vi "powermeter-medir.vi"(8 "error in (no error)":errorcluster, 11 "Powermeter":refnum<vi>) -> (0 "error out":errorcluster)   [LabVIEW 2016]
uses:
  controls/powermeter.ctl
  <vilib>/Analysis/NI_AALBase.lvlib
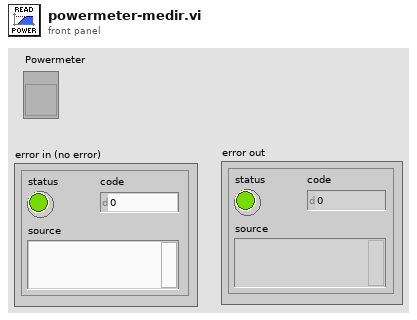
[diagram p1: front panel]
types:
  T1 = typedef "powermeter.ctl" = cluster{"Start":bool, "Serial ":string, "Model":string, "Sensor":string, "Power":dbl, "Density":bool, "Lambda":dbl, "Open":bool, "Save":bool, "reference":refnum<k7>, "hDevice":i32, "Dev. Std.":dbl, "Channel":i16}
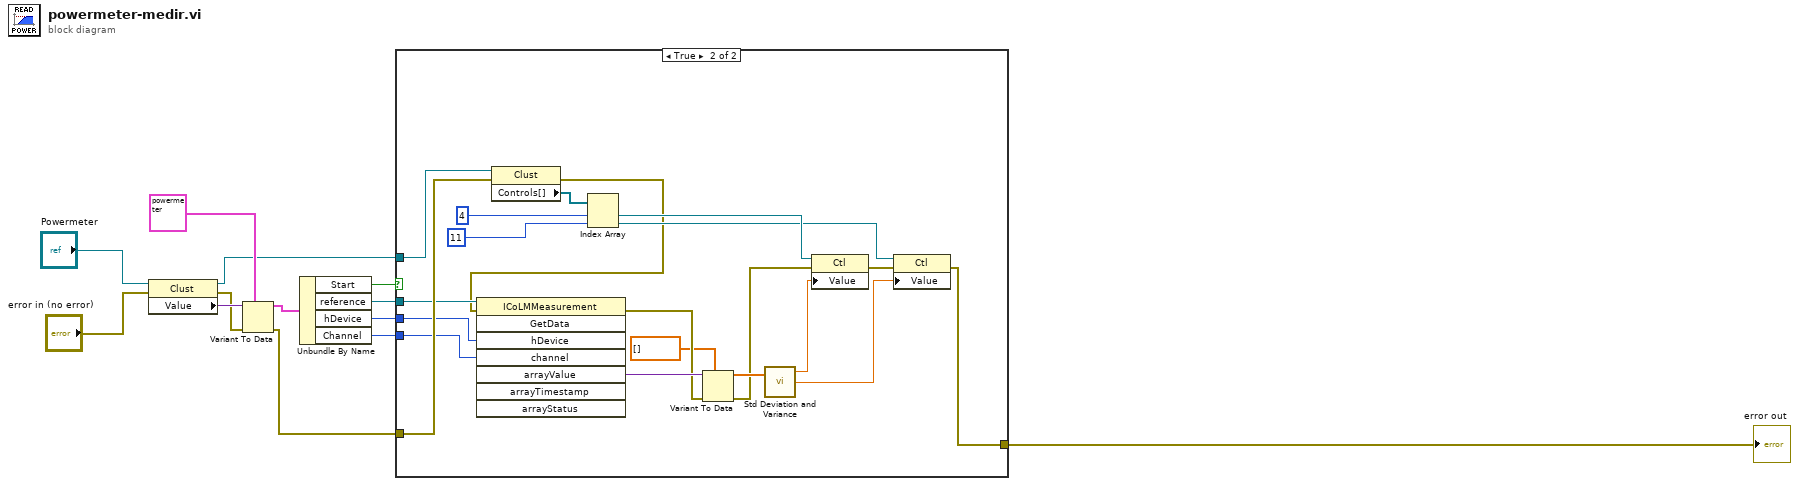
[diagram p0: block diagram]
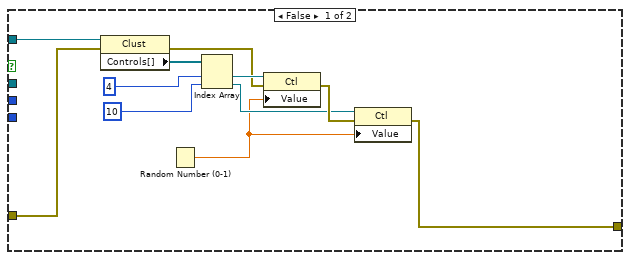
[diagram p2: hidden frame]
diagram:
  n1 = property class="Clust"(reference="Powermeter", error in="error in (no error)") -> (reference out=w4:refnum<vi>, error out=w8:errorcluster, "Value"=w9:variant)
  n2 = Variant To Data(error in=w8, type=T1 {"Start"=FALSE, "Serial "="", "Model"="", "Sensor"="", "Power"=0.0, "Density"=FALSE, "Lambda"=0.0, "Open"=FALSE, "Save"=FALSE, "reference"=refnum, "hDevice"=0, "Dev. Std."=0.0, "Channel"=0} ("Power Meter in"), Variant=w9) -> (data=w6:T1, error out=w5:errorcluster)
  n3 = Unbundle By Name(w6) -> ("Start"=w12:bool, "reference"=w3:refnum<k7>, "hDevice"=w2:i32, "Channel"=w1:i16)
  n4 = case shown="True" w12 {
    tunnel: [w14 w25] -> w13
    tunnel: w5 -> [w24 w41]
    tunnel: w4 -> [w23 w42]
    tunnel: w3 -> [_ w38]
    tunnel: w2 -> [_ w37]
    tunnel: w1 -> [_ w36]
    frame False {
      n5 = property class="Clust"(reference=w23, error in=w24) -> (error out=w18:errorcluster, "Controls[]"=w22:refnum<vi>[])  [unwired: 1 out]
      n6 = Random Number (0-1)() -> (number: 0 to 1=w15:dbl)
      n7 = Index Array(array=w22, index #1=4 ("index"), index #2=10 ("index")) -> (element #1=w19:refnum<vi>, element #2=w16:refnum<vi>)
      n8 = property class="Ctl"(reference=w19, error in=w18, "Value"=w15) -> (error out=w17:errorcluster)  [unwired: 1 out]
      n9 = property class="Ctl"(reference=w16, error in=w17, "Value"=w15) -> (error out=w14:errorcluster)  [unwired: 1 out]
    }
    frame True {
      n10 = property class="Clust"(reference=w42, error in=w41) -> (error out=w28:errorcluster, "Controls[]"=w40:refnum<vi>[])  [unwired: 1 out]
      n11 = invoke class="ICoLMMeasurement" method="GetData"(reference=w38, error in=w28, "hDevice"=w37, "channel"=w36) -> (error out=w31:errorcluster, "arrayValue"=w44:variant)  [unwired: 4 in, 6 out]
      n12 = Index Array(array=w40, index #1=4 ("index"), index #2=11 ("index")) -> (element #1=w35:refnum<vi>, element #2=w32:refnum<vi>)
      n13 = Variant To Data(error in=w31, type=dbl[] [], Variant=w44) -> (data=w43:dbl[], error out=w30:errorcluster)
      n14 = call <vilib>:"Std Deviation and Variance.vi"("X"=w43) -> ("mean"=w27:dbl, "standard deviation"=w26:dbl)  [unwired: 1 in, 1 out]
      n15 = property class="Ctl"(reference=w35, error in=w30, "Value"=w27) -> (error out=w33:errorcluster)  [unwired: 1 out]
      n16 = property class="Ctl"(reference=w32, error in=w33, "Value"=w26) -> (error out=w25:errorcluster)  [unwired: 1 out]
    }
  }
  "error out" <- w13
